vi "Reset old test Values (SubVI) Kinetics.vi"(8 "error in":errorcluster, 9 "Atr in":refnum<vi>, 11 "Test Paragraph":string) -> (0 "error out":errorcluster, 1 "Atr out":refnum<vi>, 3 "Atr Out":string[][](array[string]))   [LabVIEW 2017]
uses:
  <vilib>/Utility/miscctls.llb/LVRowAndColumnTypeDef.ctl
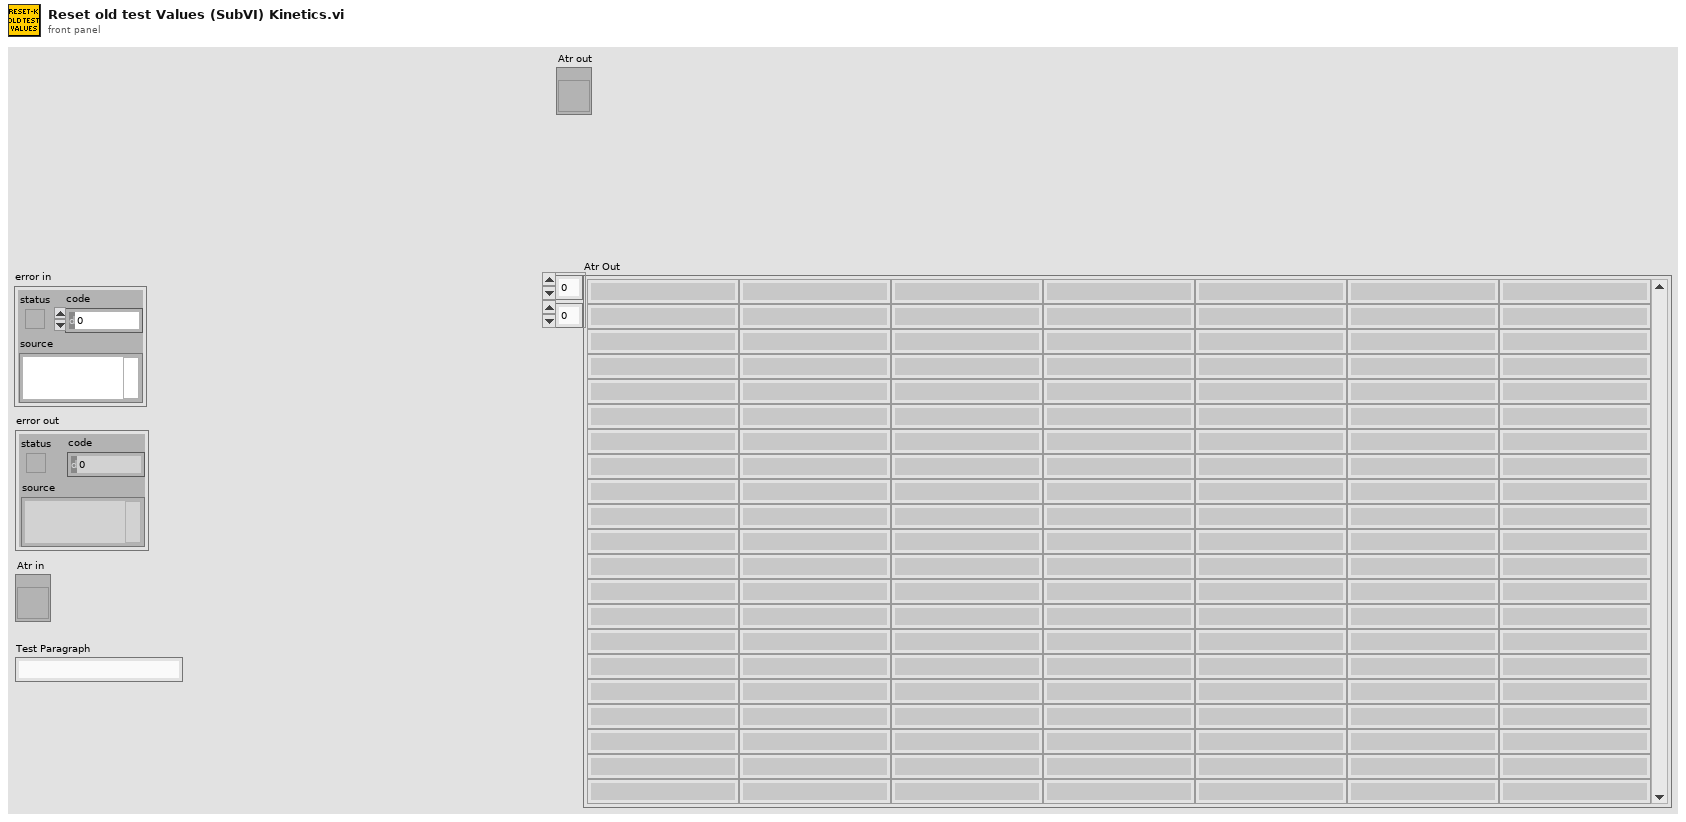
[diagram p1: front panel]
types:
  T1 = typedef "LVRowAndColumnTypeDef.ctl" = cluster{"Row":i32, "Column":i32}
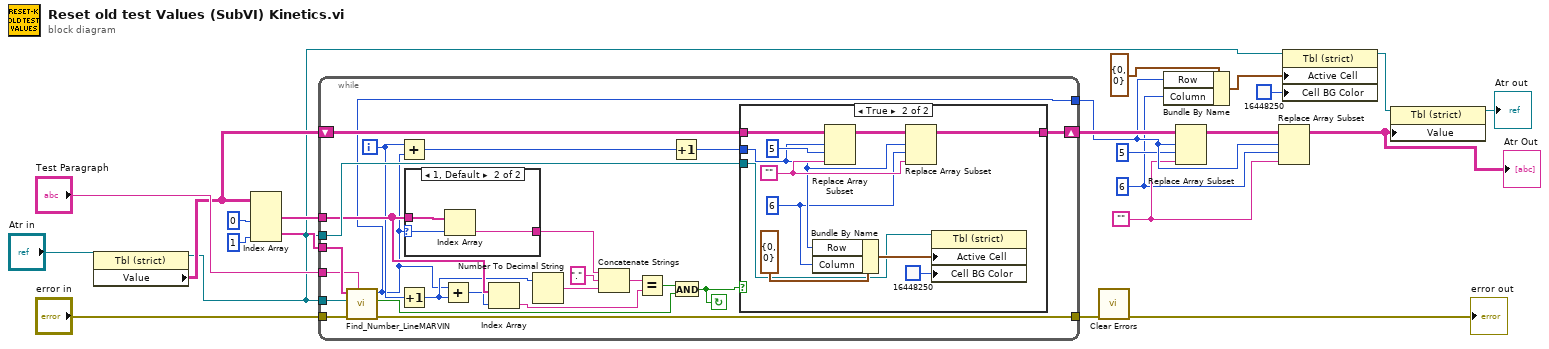
[diagram p0: block diagram]
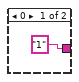
[diagram p2: hidden frame]
diagram:
  w9 = ""
  w6 = 6 ("disabled index (col)")
  n1 = property class="Tbl (strict)"(reference="Atr in") -> (reference out=w13:refnum<vi>, "Value"=w15:string[][])  [unwired: 1 in, 1 out]
  n2 = Index Array(array=w15, index (col) #1=0 ("disabled index (col)"), index (col) #2=1 ("disabled index (col)")) -> (element #1=w16:string[], element #2=w18:string[])  [unwired: 2 in]
  n3 = while {
    tunnel: w18 -> [w46]
    tunnel: "Test Paragraph" -> [w39]
    tunnel: "error in" -> [w45]
    tunnel: [w44] -> w22
    shift-right: [w43] -> w14
    shift-left: w15 -> [w42]
    tunnel: w13 -> [w41]
    tunnel: w13 -> [w40]
    tunnel: w16 -> [w36]
    tunnel: [w24] -> w12
    i -> [w29]
    stop <- w33 continue-if-true
    n4 = call "Find_Number_LineMARVIN.vi"("Test Paragraph"=w39, "error in"=w45, "TableIn"=w40, "Row Headers[]"=w46) -> ("error out"=w44:errorcluster, "Found"=w35:bool, "Line number"=w24:i32)  [unwired: 1 in, 1 out]
    n5 = Add(x=w29, y=w24) -> (x+y=w34:i32)
    n6 = Increment(x=w29) -> (x+1=w26:i32)
    n7 = case shown="1, Default" w24 {
      selector: w24 -> [_ w48]
      tunnel: w36 -> [_ w50]
      tunnel: ["1" w49] -> w27
      frame 0 {
      }
      frame 1, Default {
        n8 = Index Array(array=w50, index=w48) -> (element=w49:string)
      }
    }
    n9 = Add(x=w24, y=w26) -> (x+y=w30:i32)
    n10 = Index Array(array=w36, index=w30) -> (element=w32:string)
    n11 = Number To Decimal String(number=w26) -> (decimal integer string=w38:string)  [unwired: 1 in]
    n12 = Concatenate Strings(w27, "." ("string"), w38) -> (w31:string)
    n13 = Equal?(x=w31, y=w32) -> (x = y?=w28:bool)
    n14 = Increment(x=w34) -> (x+1=w25:i32)
    n15 = And(x=w28, y=w35) -> (x .and. y?=w33:bool)
    n16 = case shown="True" w33 {
      tunnel: [w51 w61] -> w43
      tunnel: w42 -> [w51 w60]
      tunnel: w25 -> [_ w55]
      tunnel: w41 -> [_ w52]
      frame False {
      }
      frame True {
        w58 = ""
        w54 = 6 ("disabled index (col)")
        n17 = Bundle By Name(cluster=T1 {"Row"=0, "Column"=0} ("Active Cell:Active Cell"), "Row"=w55, "Column"=w54) -> (w57:T1)
        n18 = Replace Array Subset(array=w60, new element=w58, index (row)=w55, index (col)=5 ("disabled index (col)")) -> (w62:string[][])
        n19 = Replace Array Subset(array=w62, new element=w58, index (row)=w55, index (col)=w54) -> (w61:string[][])
        n20 = property class="Tbl (strict)"(reference=w52, "Active Cell"=w57, "Cell BG Color"=u32 16448250) -> ()  [unwired: 1 in, 2 out]
      }
    }
  }
  n21 = call <vilib>:"Clear Errors.vi"("error in (no error)"=w22) -> ("error out"=→"error out":errorcluster)  [unwired: 5 in, 1 out]
  n22 = Bundle By Name(cluster=T1 {"Row"=0, "Column"=0} ("Active Cell:Active Cell"), "Row"=w12, "Column"=w6) -> (w8:T1)
  n23 = Replace Array Subset(array=w14, new element=w9, index (row)=w12, index (col)=5 ("disabled index (col)")) -> (w11:string[][])
  n24 = Replace Array Subset(array=w11, new element=w9, index (row)=w12, index (col)=w6) -> (w1:string[][])
  "Atr Out" <- w1
  n25 = property class="Tbl (strict)"(reference=w13, "Active Cell"=w8, "Cell BG Color"=u32 16448250) -> (reference out=w4:refnum<vi>)  [unwired: 1 in, 1 out]
  n26 = property class="Tbl (strict)"(reference=w4, "Value"=w1) -> (reference out=→"Atr out":refnum<vi>)  [unwired: 1 in, 1 out]
